vi "Sort_Tracks_with_and_without_Problems-4.vi"(6 "error IN":errorcluster, 8 "[IN] Dot matrix":i16[][](array[numeric]), 9 "[IN}Frame-to-frame displ":dbl[][](array[numeric])) -> (0 "error OUT":errorcluster, 1 "[OUT] Imaging (Tracks w/t problems)":dbl[][](array[numeric]), 3 "[OUT] Tracks w/t Problems":T1(array[cluster]), 4 "[OUT] Filtered Dot Matrix":i16[][](array[numeric]), 5 "[OUT] Displacements with problems\nCollected in Columns (as raw displ)":dbl[][](array[numeric]))   [LabVIEW 2017]
doc: "SubVI makes and separates after it the tracks to the group with problems and to the group without any problems"
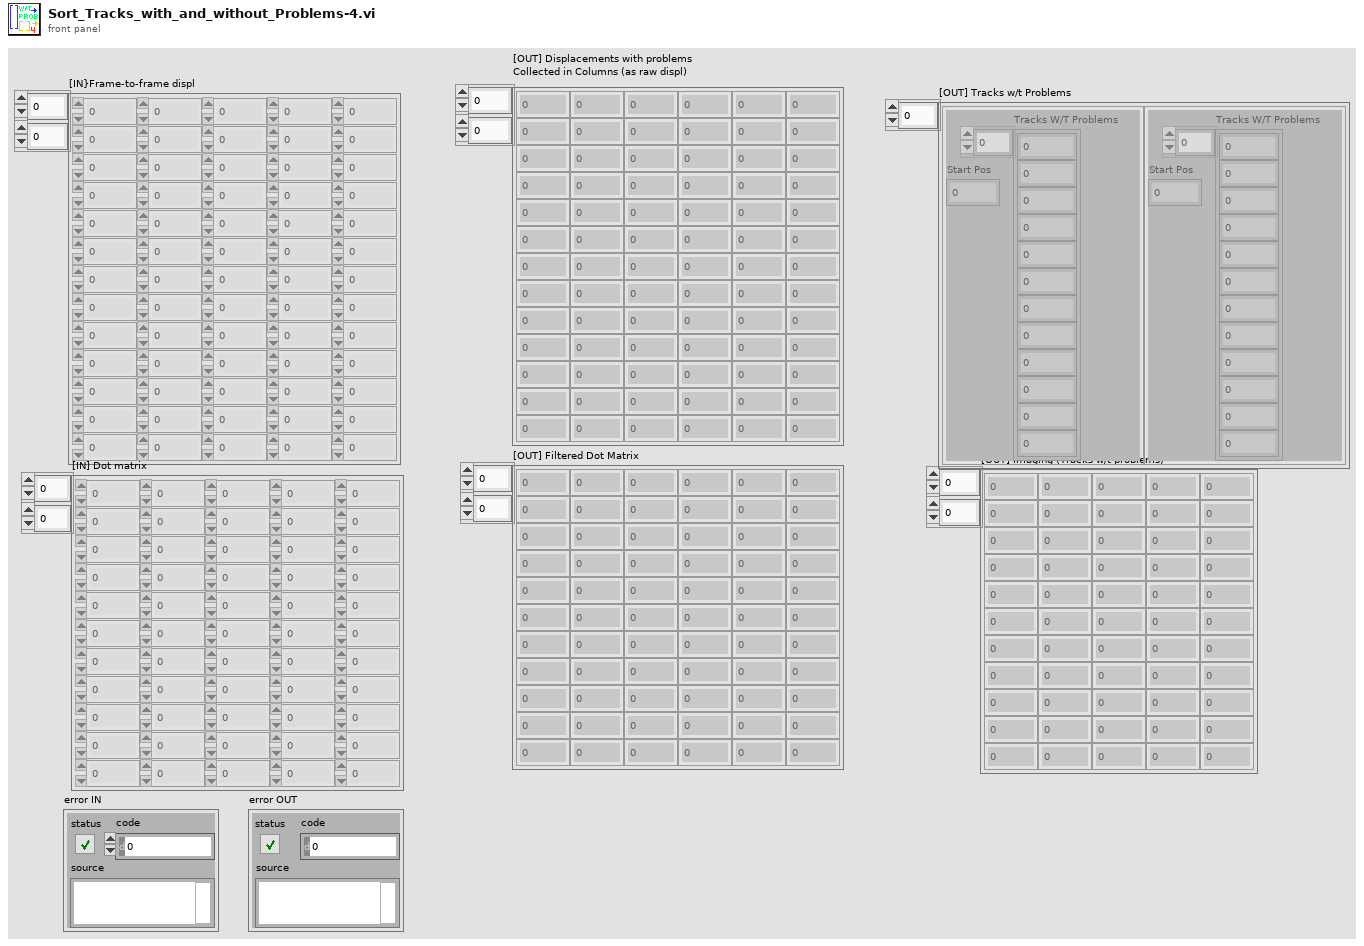
[diagram p1: front panel]
types:
  T1 = cluster{"Tracks W/T Problems":dbl[], "Start Pos":i32}[]
  T2 = cluster{"Tracks W/T Problems":dbl[], "Start Pos":i32}
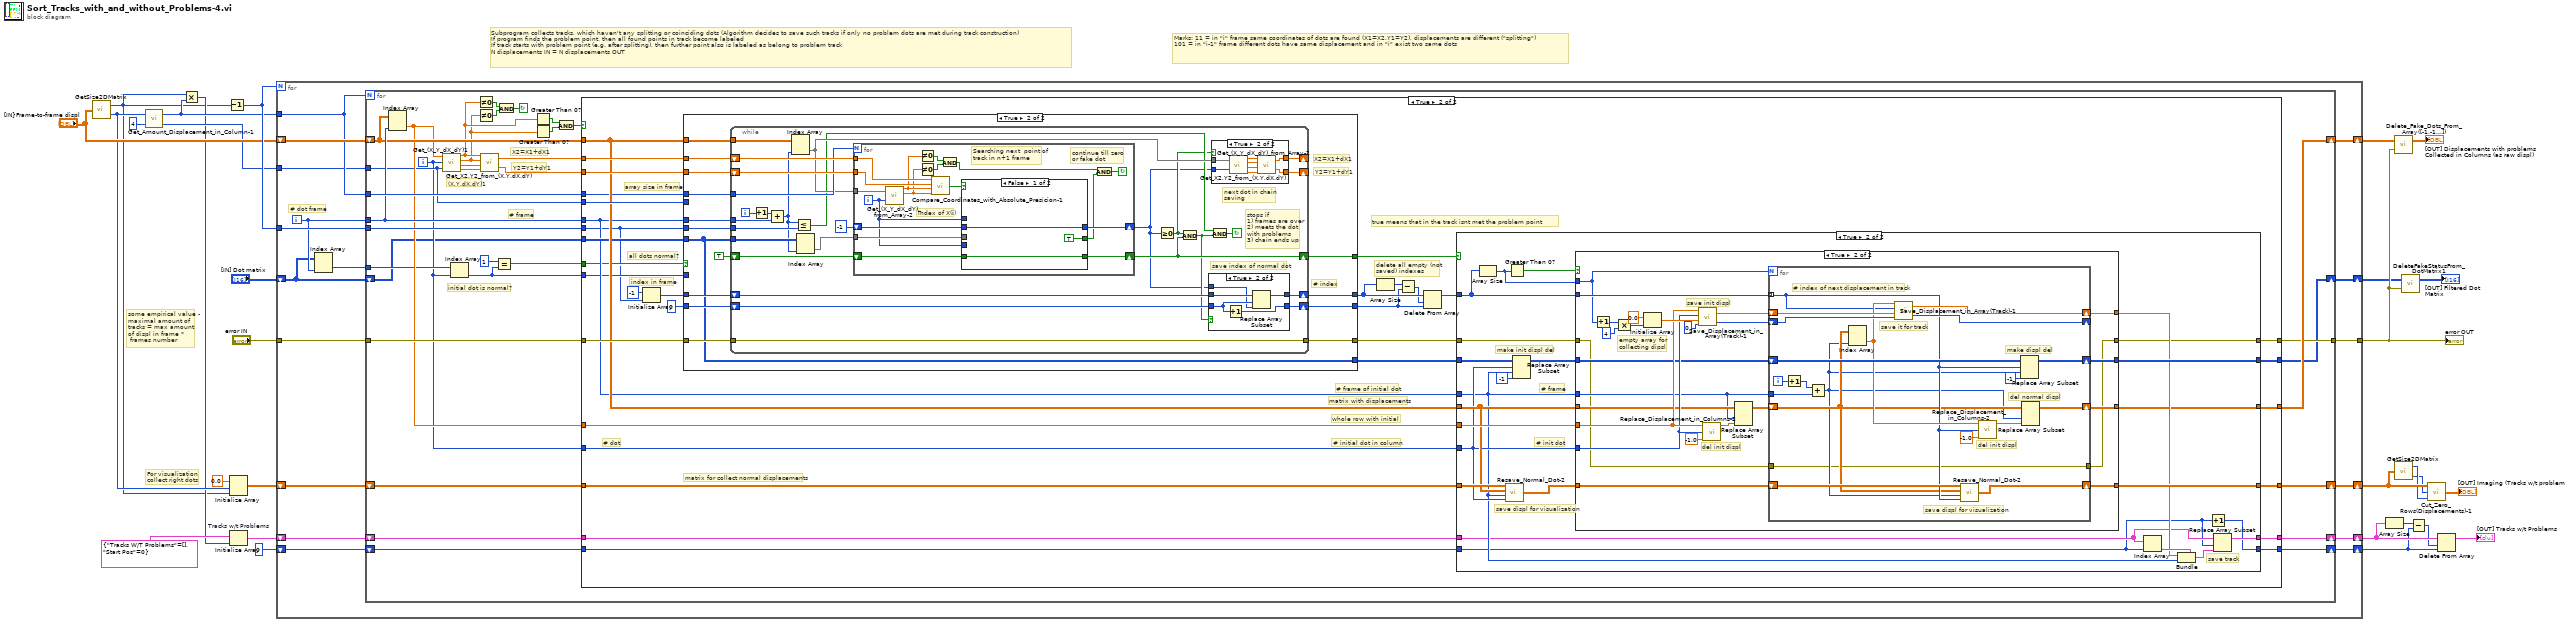
[diagram p0: block diagram]
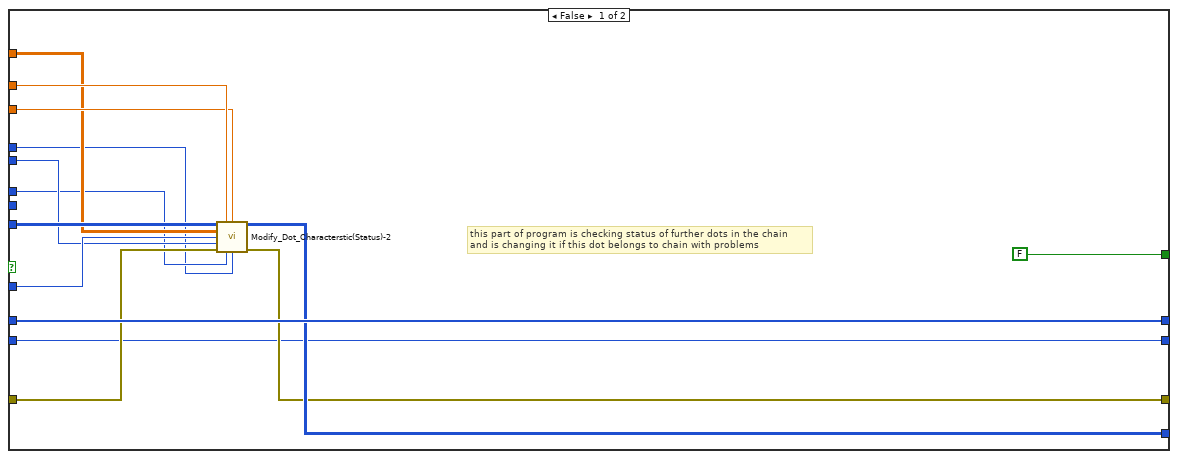
[diagram p3: hidden frame]
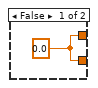
[diagram p4: hidden frame]
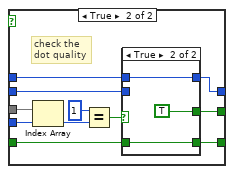
[diagram p6: hidden frame]
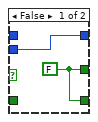
[diagram p7: hidden frame]
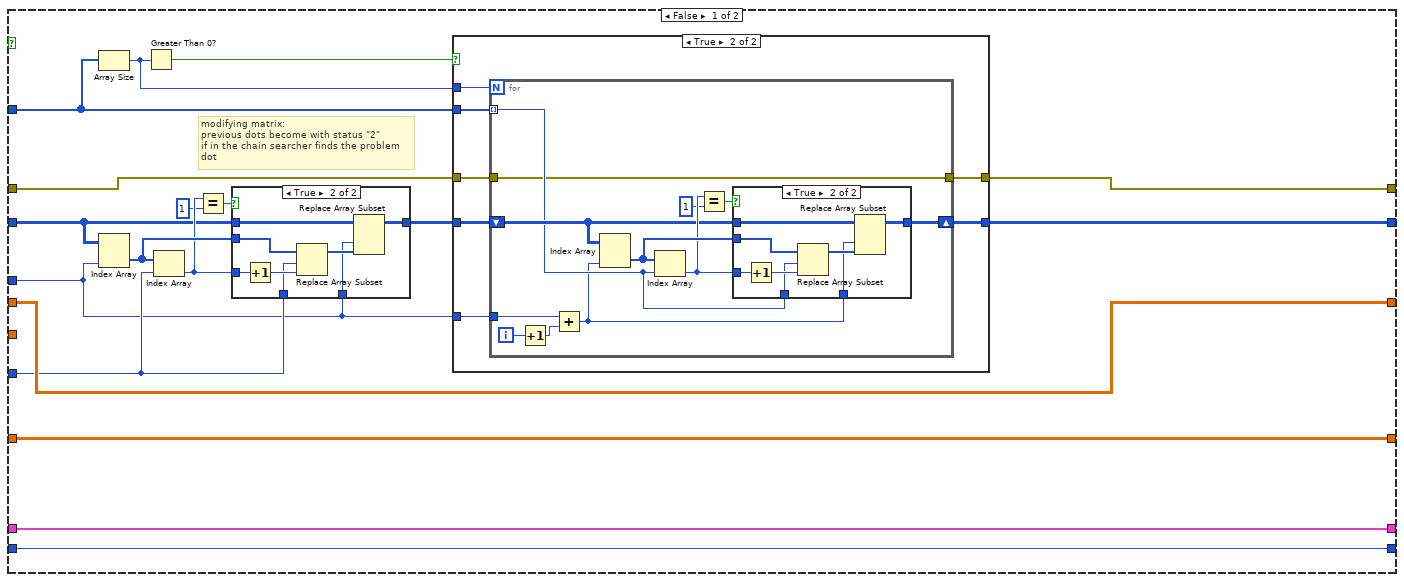
[diagram p8: hidden frame]
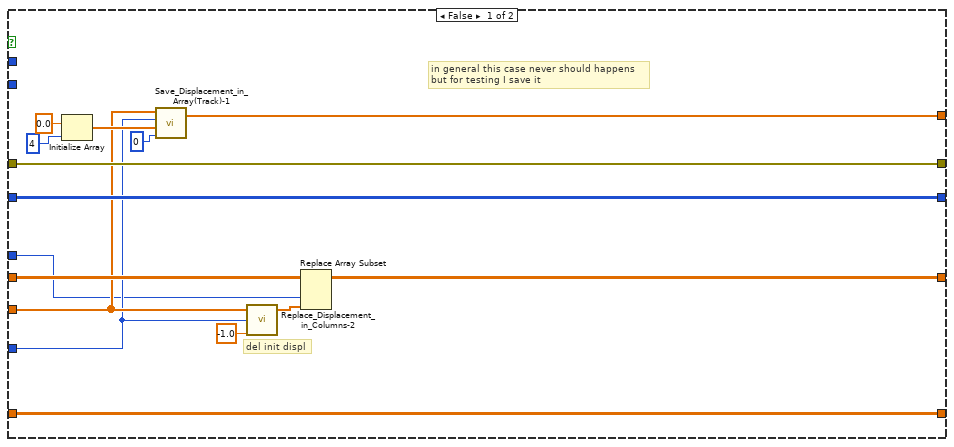
[diagram p12: hidden frame]
diagram:
  # "some empirical value -\nmaximal amount of\ntracks = max amount \nof displ in frame * \n frames number"
  # "For visualization\ncollect right dots"
  # "Marks: 11 = in \"i\" frame same coordinates of dots are found (X1=X2,Y1=Y2), displacements are different (\"splitting\")\n101 = in \"i-1\" frame different dots have same displacement and in \"i\" exist two same dots"
  # "Subprogram collects tracks, which haven't any splitting or coinciding dots (Algorithm decides to save such tracks if only no problem dots are met during track construction)\nIf program finds the problem point, then all found points in track become labeled\nIf track starts with problem point (e.g. after splitting), then further point also is labeled as belong to problem track\nN displacements IN = N displacements OUT"
  n1 = call "GetSize2DMatrix.vi"("Array IN (2D)"="[IN}Frame-to-frame displ") -> ("# Cols"=w7:i32, "# Rows"=w15:i32)
  n2 = call "Get_Amount_Displacement_in_Column-1.vi"("multiplier"=4 ("y"), "# Rows"=w15) -> ("multiplier out"=w12:i32, "Displ amount"=w13:i32)
  n3 = Multiply(x=w7, y=w13) -> (x*y=w10:i32)
  n4 = Decrement(x=w7) -> (x-1=w29:i32)
  n5 = Initialize Array(0.0 ("element"), w15, w7) -> (w27:dbl[][])
  n6 = Initialize Array "Tracks w/t Problems"(T2 {"Tracks W/T Problems"=[], "Start Pos"=0} ("element"), w10) -> (w9:T1)
  n7 = for {
    N: w29 -> [_]
    shift-right: [w43] -> w18
    shift-left: "[IN}Frame-to-frame displ" -> [w46]
    tunnel: w29 -> [w45]
    tunnel: "error IN" -> [w44]
    tunnel: [w42] -> w22
    shift-right: [w38] -> w26
    shift-left: w27 -> [w39]
    shift-right: [w36] -> w17
    shift-left: "[IN] Dot matrix" -> [w37]
    tunnel: w13 -> [w35]
    tunnel: w12 -> [w34]
    shift-right: [w31] -> w5
    shift-left: w9 -> [w33]
    shift-right: [w30] -> w3
    shift-left: 0 -> [w32]
    i -> [w41]
    # "# dot frame"
    n8 = Index Array(array=w37, index (col)=w41) -> (element=w40:i16[])  [unwired: 1 in]
    n9 = for {
      N: w35 -> [_]
      tunnel: w34 -> [w69]
      tunnel: w41 -> [w72]
      tunnel: w35 -> [w77]
      shift-right: [w74] -> w43
      shift-left: w46 -> [w71]
      tunnel: w45 -> [w76]
      tunnel: w44 -> [w75]
      tunnel: [w73] -> w42
      tunnel: w40 -> [w65]
      shift-right: [w59] -> w38
      shift-left: w39 -> [w60]
      shift-right: [w57] -> w36
      shift-left: w37 -> [w58]
      shift-right: [w48] -> w31
      shift-left: w33 -> [w50]
      shift-right: [w47] -> w30
      shift-left: w32 -> [w49]
      i -> [w64]
      stop <- w78 continue-if-true
      # "initial dot is normal?"
      # "# frame"
      # "Y2=Y1+dY1"
      # "X2=X1+dX1"
      # "(X,Y,dX,dY)1"
      n10 = Index Array(array=w71, index (col)=w72) -> (element=w70:dbl[])  [unwired: 1 in]
      n11 = call "Get_(X_Y_dX_dY)1.vi"("(X,Y,dX,dY)"=w70, "index"=w64, "multiplier"=w69) -> ("X"=w56:dbl, "Y"=w55:dbl, "dX"=w53:dbl, "dY"=w52:dbl)
      n12 = Index Array(array=w65, index=w64) -> (element=w61:i16)
      n13 = Not Equal To 0?(x=w56) -> (x != 0?=w80:bool)
      n14 = Not Equal To 0?(x=w55) -> (x != 0?=w79:bool)
      n15 = call "Get_X2,Y2_from_(X,Y,dX,dY).vi"("dY"=w52, "dX"=w53, "Y1"=w55, "X1"=w56) -> ("Y2 = (Y1+dY)"=w51:dbl, "X2 = (X1+dX)"=w54:dbl)
      n16 = Equal?(x=i16 1, y=w61) -> (x = y?=w62:bool)
      n17 = And(x=w80, y=w79) -> (x .and. y?=w78:bool)
      n18 = Greater Than 0?(x=w56) -> (x > 0?=w68:bool)
      n19 = Greater Than 0?(x=w55) -> (x > 0?=w67:bool)
      n20 = And(x=w68, y=w67) -> (x .and. y?=w63:bool)
      n21 = case shown="True" w63 {
        tunnel: w71 -> [w86 w113]
        tunnel: w54 -> [_ w119]
        tunnel: w51 -> [_ w118]
        tunnel: w72 -> [_ w108]
        tunnel: w77 -> [_ w100]
        tunnel: w69 -> [_ w117]
        tunnel: w76 -> [_ w99]
        tunnel: w75 -> [w85 w116]
        tunnel: w70 -> [_ w112]
        tunnel: [w86 w114] -> w74
        tunnel: [w85 w115] -> w73
        tunnel: w58 -> [w84 w109]
        tunnel: w64 -> [_ w107]
        tunnel: [w84 w106] -> w57
        tunnel: w62 -> [_ w105]
        tunnel: w61 -> [_ w104]
        tunnel: w60 -> [w83 w98]
        tunnel: [w83 w97] -> w59
        tunnel: w50 -> [w82 w95]
        tunnel: w49 -> [w81 w94]
        tunnel: [w82 w88] -> w48
        tunnel: [w81 w87] -> w47
        frame False {
        }
        frame True {
          # "matrix with displacements"
          # "# initial dot in column"
          # "# frame of initial dot"
          # "delete all empty (not \nsaved) indexes"
          # "true means that in the track isnt met the problem point"
          # "whole row with initial"
          # "# dot"
          # "matrix for collect normal displacements"
          # "all dots normal?"
          # "array size in frame"
          # "index in frame"
          n22 = Initialize Array(-1 ("element"), w99) -> (w101:i32[])
          n23 = case shown="True" w105 {
            tunnel: w119 -> [w131 w148]
            tunnel: w118 -> [w130 w147]
            tunnel: w99 -> [_ w146]
            tunnel: w117 -> [w124 _]
            tunnel: w116 -> [w123 w145]
            tunnel: [w133 w144] -> w93
            tunnel: w100 -> [w121 w143]
            tunnel: w113 -> [w126 w142]
            tunnel: [FALSE w140] -> w111
            tunnel: [w128 w139] -> w110
            tunnel: w109 -> [w127 w135]
            tunnel: w108 -> [w122 w138]
            tunnel: w104 -> [w125 _]
            tunnel: 0 -> [w120 w137]
            tunnel: w101 -> [w133 w136]
            tunnel: [w129 w135] -> w96
            tunnel: [w120 w134] -> w91
            frame False {
              # "this part of program is checking status of further dots in the chain\nand is changing it if this dot belongs to chain with problems"
              n24 = call "Modify_Dot_Characterstic(Status)-2.vi"("Dot matrix IN"=w127, "X2"=w131, "Y2"=w130, "Frame-to-frame displ"=w126, "Dot charact"=w125, "multipler"=w124, "error IN"=w123, "# column"=w122, "Size Rows"=w121) -> ("Dot matrix OUT"=w129:i16[][], "error OUT"=w128:errorcluster)  [unwired: 5 in]
            }
            frame True {
              # "Y2=Y1+dY1"
              # "X2=X1+dX1"
              # "# index"
              n25 = while {
                tunnel: w146 -> [w161]
                tunnel: w138 -> [w171]
                tunnel: w143 -> [w168]
                shift-right: [w165] -> w144
                shift-left: w136 -> [w167]
                shift-right: [w164] -> w134
                shift-left: w137 -> [w166]
                tunnel: w142 -> [w170]
                tunnel: w145 -> [w162]
                tunnel: [w162] -> w139
                shift-right: [w159] -> _
                shift-left: w148 -> [w173]
                shift-right: [w158] -> _
                shift-left: w147 -> [w172]
                tunnel: w135 -> [w157]
                shift-right: [w151] -> w140
                shift-left: TRUE -> [w154]
                i -> [w175]
                stop <- w163 continue-if-true
                # "stops if \n1) frames are over\n2) meets the dot \nwith problems\n3) chain ends up"
                # "next dot in chain\nsaving"
                # "save index of normal dot"
                n26 = Increment(x=w175) -> (x+1=w174:i32)
                n27 = Add(x=w174, y=w171) -> (x+y=w156:i32)
                n28 = Index Array(array=w170, index (col)=w156) -> (element=w160:dbl[])  [unwired: 1 in]
                n29 = Less Or Equal?(x=w156, y=w161) -> (x <= y?=w153:bool)
                n30 = Index Array(array=w157, index (col)=w156) -> (element=w155:i16[])  [unwired: 1 in]
                n31 = for {
                  N: w168 -> [_]
                  tunnel: w160 -> [w195]
                  tunnel: w173 -> [w198]
                  tunnel: w172 -> [w197]
                  shift-right: [w205] -> w149
                  shift-left: -1 -> [w206]
                  tunnel: w155 -> [w204]
                  shift-right: [w199] -> w151
                  shift-left: w154 -> [w200]
                  i -> [w194]
                  stop <- w201 continue-if-true
                  # "continue till zero\nor fake dot"
                  # "Searching next  point of track in n+1 frame"
                  # "index of X(i)"
                  n32 = call "Get_(X_Y_dX_dY)_from_Array-2.vi"("(X,Y,dX,dY)"=w195, "Index of Displacement"=w194) -> ("X"=w193:dbl, "Y"=w192:dbl)  [unwired: 2 out]
                  n33 = Not Equal To 0?(x=w193) -> (x != 0?=w208:bool)
                  n34 = Not Equal To 0?(x=w192) -> (x != 0?=w207:bool)
                  n35 = call "Compare_Coordinates_with_Absolute_Presicion-1.vi"("X 1"=w198, "Y 1"=w197, "X 2"=w193, "Y 2"=w192) -> ("[OUT] Same coordinates?"=w196:bool)  [unwired: 1 in]
                  n36 = And(x=w208, y=w207) -> (x .and. y?=w202:bool)
                  n37 = case shown="False" w196 {
                    tunnel: w194 -> [_ w217]
                    tunnel: w206 -> [w211 w215]
                    tunnel: [w211 w216] -> w205
                    tunnel: w204 -> [_ w222]
                    tunnel: w194 -> [_ w221]
                    tunnel: [TRUE w214] -> w203
                    tunnel: w200 -> [w209 w213]
                    tunnel: [w209 w212] -> w199
                    frame False {
                    }
                    frame True {
                      # "check the \ndot quality"
                      n38 = Index Array(array=w222, index=w221) -> (element=w219:i16)
                      n39 = Equal?(x=i16 1, y=w219) -> (x = y?=w218:bool)
                      n40 = case shown="True" w218 {
                        tunnel: [w224 w227] -> w216
                        tunnel: w217 -> [_ w227]
                        tunnel: w215 -> [w224 _]
                        tunnel: [w223 TRUE] -> w214
                        tunnel: w213 -> [_ w225]
                        tunnel: [w223 w225] -> w212
                        frame False {
                          w223 = FALSE
                        }
                        frame True {
                        }
                      }
                    }
                  }
                  n41 = And(x=w202, y=w203) -> (x .and. y?=w201:bool)
                }
                n42 = Greater Or Equal To 0?(x=w149) -> (x >= 0?=w152:bool)
                n43 = And(x=w152, y=w151) -> (x .and. y?=w150:bool)
                n44 = case shown="True" w150 {
                  tunnel: w167 -> [w186 w191]
                  tunnel: w166 -> [w185 w190]
                  tunnel: [w186 w189] -> w165
                  tunnel: [w185 w188] -> w164
                  tunnel: w149 -> [_ w187]
                  frame False {
                  }
                  frame True {
                    n45 = Increment(x=w190) -> (x+1=w188:i32)
                    n46 = Replace Array Subset(array=w191, new element=w187, index=w190) -> (w189:i32[])
                  }
                }
                n47 = case shown="True" w152 {
                  tunnel: w160 -> [_ w181]
                  tunnel: [w176 w184] -> w159
                  tunnel: [w176 w183] -> w158
                  tunnel: w149 -> [_ w182]
                  frame False {
                    w176 = 0.0
                  }
                  frame True {
                    n48 = call "Get_(X_Y_dX_dY)_from_Array-2.vi"("(X,Y,dX,dY)"=w181, "Index of Displacement"=w182) -> ("X"=w180:dbl, "Y"=w179:dbl, "dX"=w178:dbl, "dY"=w177:dbl)
                    n49 = call "Get_X2,Y2_from_(X,Y,dX,dY).vi"("dY"=w177, "dX"=w178, "Y1"=w179, "X1"=w180) -> ("Y2 = (Y1+dY)"=w183:dbl, "X2 = (X1+dX)"=w184:dbl)
                  }
                }
                n50 = And(x=w153, y=w150) -> (x .and. y?=w163:bool)
              }
            }
          }
          n51 = Array Size(array=w93) -> (size(s)=w92:i32)
          n52 = Subtract(x=w92, y=w91) -> (x-y=w90:i32)
          n53 = Delete From Array(array=w93, length=w90, index=w91) -> (array with subset deleted=w89:i32[])  [unwired: 1 out]
          n54 = case shown="True" w111 {
            tunnel: w110 -> [w231 w286]
            tunnel: w112 -> [_ w300]
            tunnel: w108 -> [w232 w293]
            tunnel: w113 -> [w245 w299]
            tunnel: [w245 w287] -> w114
            tunnel: [w230 w285] -> w115
            tunnel: w96 -> [w240 w307]
            tunnel: w107 -> [w239 w298]
            tunnel: [w235 w296] -> w106
            tunnel: w98 -> [w238 w308]
            tunnel: [w238 w297] -> w97
            tunnel: w95 -> [w229 w292]
            tunnel: w94 -> [w228 w289]
            tunnel: w89 -> [w233 w304]
            tunnel: [w229 w290] -> w88
            tunnel: [w228 w288] -> w87
            frame False {
              # "modifying matrix: \nprevious dots become with status \"2\" \nif in the chain searcher finds the problem\ndot"
              n55 = Array Size(array=w233) -> (size(s)=w234:i32)
              n56 = Index Array(array=w240, index (col)=w232) -> (element=w244:i16[])  [unwired: 1 in]
              n57 = Greater Than 0?(x=w234) -> (x > 0?=w237:bool)
              n58 = Index Array(array=w244, index=w239) -> (element=w243:i16)
              n59 = Equal?(x=w243, y=i16 1) -> (x = y?=w242:bool)
              n60 = case shown="True" w242 {
                tunnel: w243 -> [_ w284]
                tunnel: w244 -> [_ w283]
                tunnel: w239 -> [_ w281]
                tunnel: w240 -> [w276 w280]
                tunnel: [w276 w278] -> w236
                tunnel: w232 -> [_ w277]
                frame False {
                }
                frame True {
                  n61 = Increment(x=w284) -> (x+1=w282:i16)
                  n62 = Replace Array Subset(array=w283, new element=w282, index=w281) -> (w279:i16[])
                  n63 = Replace Array Subset(array=w280, new element=w279, index (col)=w277) -> (w278:i16[][])  [unwired: 1 in]
                }
              }
              n64 = case shown="True" w237 {
                tunnel: w236 -> [w247 w252]
                tunnel: [w247 w251] -> w235
                tunnel: w234 -> [_ w254]
                tunnel: w233 -> [_ w253]
                tunnel: w232 -> [_ w250]
                tunnel: w231 -> [w246 w249]
                tunnel: [w246 w248] -> w230
                frame False {
                }
                frame True {
                  n65 = for {
                    N: w254 -> [_]
                    tunnel: w253 -> [w258] mode=indexing
                    shift-right: [w256] -> w251
                    shift-left: w252 -> [w259]
                    tunnel: w250 -> [w261]
                    tunnel: w249 -> [w255]
                    tunnel: [w255] -> w248
                    i -> [w262]
                    n66 = Increment(x=w262) -> (x+1=w260:i32)
                    n67 = Add(x=w261, y=w260) -> (x+y=w257:i32)
                    n68 = Index Array(array=w259, index (col)=w257) -> (element=w266:i16[])  [unwired: 1 in]
                    n69 = Index Array(array=w266, index=w258) -> (element=w265:i16)
                    n70 = Equal?(x=w265, y=i16 1) -> (x = y?=w264:bool)
                    n71 = case shown="True" w264 {
                      tunnel: w265 -> [_ w275]
                      tunnel: w266 -> [_ w274]
                      tunnel: w258 -> [_ w272]
                      tunnel: w259 -> [w267 w271]
                      tunnel: [w267 w269] -> w256
                      tunnel: w257 -> [_ w268]
                      frame False {
                      }
                      frame True {
                        n72 = Increment(x=w275) -> (x+1=w273:i16)
                        n73 = Replace Array Subset(array=w274, new element=w273, index=w272) -> (w270:i16[])
                        n74 = Replace Array Subset(array=w271, new element=w270, index (col)=w268) -> (w269:i16[][])  [unwired: 1 in]
                      }
                    }
                  }
                }
              }
            }
            frame True {
              # "save track"
              # "save displ for visualization"
              # "# init dot"
              # "# frame"
              # "make init displ del"
              n75 = Array Size(array=w304) -> (size(s)=w302:i32)
              n76 = call "Resave_Normal_Dot-2.vi"("starting index (dot)"=w298, "# column"=w293, "[IN] Source matrix"=w299, "[IN] Collect matrix"=w308) -> ("[OUT] Collect matrix"=w301:dbl[][])
              n77 = Greater Than 0?(x=w302) -> (x > 0?=w305:bool)
              n78 = Replace Array Subset(array=w307, new element=i16 -1 ("new element/subarray"), index (row)=w298, index (col)=w293) -> (w303:i16[][])
              n79 = case shown="True" w305 {
                tunnel: w304 -> [_ w348]
                tunnel: w303 -> [w318 w331]
                tunnel: w302 -> [_ w346]
                tunnel: w301 -> [w309 w330]
                tunnel: w293 -> [w311 w333]
                tunnel: w300 -> [w313 w337]
                tunnel: w299 -> [w314 w334]
                tunnel: w298 -> [w312 w336]
                tunnel: [w309 w329] -> w297
                tunnel: [w310 w328] -> w287
                tunnel: [w318 w327] -> w296
                tunnel: [w317 w326] -> w294
                tunnel: w286 -> [w323 w325]
                tunnel: [w323 w324] -> w285
                frame False {
                  # "in general this case never should happens\nbut for testing I save it"
                  # "del init displ"
                  n80 = Initialize Array(0.0 ("element"), 4 ("dimension size")) -> (w319:dbl[])
                  n81 = call "Save_Displacement_in_Array(Track)-1.vi"("[IN] Index for Collect"=0, "[IN] Collecting Array"=w319, "[IN] Index of displ"=w312, "[IN]Source Array"=w313) -> ("[OUT] Collecting Array"=w317:dbl[])  [unwired: 1 out]
                  n82 = call "Replace_Displacement_in_Columns-2.vi"("[IN] Value for replace"=-1.0, "[IN] Index of Displ"=w312, "[IN] Replaced Array"=w313) -> ("[OUT] Replaced Array"=w315:dbl[])  [unwired: 2 in]
                  n83 = Replace Array Subset(array=w314, new element=w315, index (col)=w311) -> (w310:dbl[][])  [unwired: 1 in]
                }
                frame True {
                  # "save init displ"
                  # "del init displ"
                  # "empty array for \ncollecting dipsl"
                  n84 = Increment(x=w346) -> (x+1=w345:i32)
                  n85 = Multiply(x=w345, y=4) -> (x*y=w343:i32)
                  n86 = Initialize Array(0.0 ("element"), w343) -> (w342:dbl[])
                  n87 = call "Save_Displacement_in_Array(Track)-1.vi"("[IN] Index for Collect"=0, "[IN] Collecting Array"=w342, "[IN] Index of displ"=w336, "[IN]Source Array"=w337) -> ("[OUT] Finish Index for Collect"=w339:i32, "[OUT] Collecting Array"=w340:dbl[])
                  n88 = call "Replace_Displacement_in_Columns-2.vi"("[IN] Value for replace"=-1.0, "[IN] Index of Displ"=w336, "[IN] Replaced Array"=w337) -> ("[OUT] Replaced Array"=w335:dbl[])  [unwired: 2 in]
                  n89 = Replace Array Subset(array=w334, new element=w335, index (col)=w333) -> (w332:dbl[][])  [unwired: 1 in]
                  n90 = for {
                    N: w346 -> [_]
                    tunnel: w348 -> [w356] mode=indexing
                    tunnel: w333 -> [w367]
                    shift-right: [w361] -> w326
                    shift-left: w340 -> [w364]
                    shift-right: [w362] -> _
                    shift-left: w339 -> [w363]
                    shift-right: [w352] -> w328
                    shift-left: w332 -> [w355]
                    shift-right: [w350] -> w327
                    shift-left: w331 -> [w365]
                    shift-right: [w351] -> w329
                    shift-left: w330 -> [w358]
                    tunnel: w325 -> [w349]
                    tunnel: [w349] -> w324
                    i -> [w368]
                    # "del normal displ"
                    # "save displ for visualization"
                    # "del init displ"
                    # "save it for track"
                    # "# index of next displacement in track"
                    # "make displ del"
                    n91 = Increment(x=w368) -> (x+1=w366:i32)
                    n92 = Add(x=w366, y=w367) -> (x+y=w354:i32)
                    n93 = Index Array(array=w355, index (col)=w354) -> (element=w357:dbl[])  [unwired: 1 in]
                    n94 = call "Save_Displacement_in_Array(Track)-1.vi"("[IN] Index for Collect"=w363, "[IN] Collecting Array"=w364, "[IN] Index of displ"=w356, "[IN]Source Array"=w357) -> ("[OUT] Finish Index for Collect"=w362:i32, "[OUT] Collecting Array"=w361:dbl[])
                    n95 = call "Resave_Normal_Dot-2.vi"("starting index (dot)"=w356, "# column"=w354, "[IN] Source matrix"=w355, "[IN] Collect matrix"=w358) -> ("[OUT] Collect matrix"=w351:dbl[][])
                    n96 = call "Replace_Displacement_in_Columns-2.vi"("[IN] Value for replace"=-1.0, "[IN] Index of Displ"=w356, "[IN] Replaced Array"=w357) -> ("[OUT] Replaced Array"=w353:dbl[])  [unwired: 2 in]
                    n97 = Replace Array Subset(array=w365, new element=i16 -1 ("new element/subarray"), index (row)=w356, index (col)=w354) -> (w350:i16[][])
                    n98 = Replace Array Subset(array=w355, new element=w353, index (col)=w354) -> (w352:dbl[][])  [unwired: 1 in]
                  }
                }
              }
              n99 = Index Array(array=w292, index=w289) -> (element=w295:T2)
              n100 = Bundle(cluster=w295, "Tracks W/T Problems"=w294, "Start Pos"=w293) -> (w291:T2)
              n101 = Increment(x=w289) -> (x+1=w288:i32)
              n102 = Replace Array Subset(array=w292, new element=w291, index=w289) -> (w290:T1)
            }
          }
        }
      }
    }
  }
  "error OUT" <- w22
  n103 = Array Size(array=w5) -> (size(s)=w4:i32)
  n104 = call "Delete_Fake_Dots_From_Array([-1,-1...]).vi"("error IN"=w22, "[IN] Source Array"=w18) -> ("[OUT] Filtered Array (X,Y,dX,dY)"=→"[OUT] Displacements with problems\nCollected in Columns (as raw displ)":dbl[][])  [unwired: 1 out]
  n105 = call "GetSize2DMatrix.vi"("Array IN (2D)"=w26) -> ("# Cols"=w25:i32, "# Rows"=w24:i32)
  n106 = call "DeleteFakeStatusFrom_DotMatrix1.vi"("error IN"=w22, "[IN] Source Matrix"=w17) -> ("[OUT] Filtered Dot Matrix"=→"[OUT] Filtered Dot Matrix":i16[][])  [unwired: 1 out]
  n107 = Subtract(x=w4, y=w3) -> (x-y=w2:i32)
  n108 = call "Cut_Zero_Rows(Displacements)-1.vi"("# Cols"=w25, "# Rows"=w24, "Array IN"=w26) -> ("Array OUT"=→"[OUT] Imaging (Tracks w/t problems)":dbl[][])
  n109 = Delete From Array(array=w5, length=w2, index=w3) -> (array with subset deleted=→"[OUT] Tracks w/t Problems":T1)  [unwired: 1 out]
